vi "Exposure-Save Data.vi"(0 "Params":T3={"Probe Mic Gain"=40.0, "Waveform"=enum."Tone", "CF (kHz)"=1.0, "BW (kHz)"=4.0, "Ear"=enum."Left", "Duration (min)"=0.0, "dB SPL"=120.0, "dB SPL (left)"=0.0}, 5 "SPL Log In":cluster{"t0":dbl, "dt (min)":dbl, "SPL":dbl[][]}, 7 "Spectrum":waveform(dbl)[](graph), 11 "error in (no error)":errorcluster, 13 "State":T2) -> (15 "error out":errorcluster)   [LabVIEW 2020]
uses:
  Typedefs/Exposure Parameters.ctl
  CFTS Main Panel SubVIs/CFTS-Experiment State.ctl
  epl-vi-lib/Utility VIs/Math VIs/LinSpace (x0-dx-npts).vi
  epl-vi-lib/Utility VIs/Array Manipulation VIs/Array-Dimensions (2D).vi
panel:
  in  "Noise Exposure Log File":T1
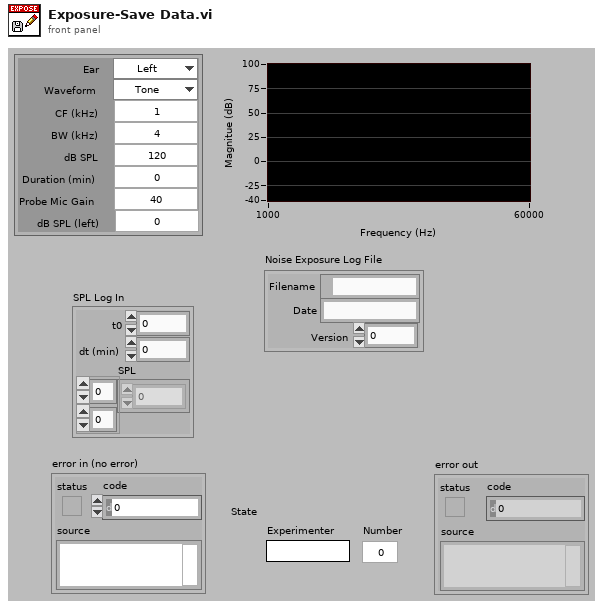
[diagram p1: front panel]
types:
  T1 = cluster{"Filename":path, "Date":string, "Version":i32}
  T2 = typedef "CFTS-Experiment State.ctl" = cluster{"Experimenter":string, "Number":u32, "Right":string, "Left":string, "Data Folder":path, "State File":path, "Version Info":string, "End Exposure Time":dbl, "Exposure Duration":string, "Run #":cluster{"CAP":i16, "ABR":i16, "DP":i16, "VsEP":i16, "MeasSeq":i16, "SubSeq":i16, "SFOAE":i16}}
  T3 = typedef "Exposure Parameters.ctl" = cluster{"Probe Mic Gain":dbl, "Waveform":enum16{"Tone", "Noise"}, "CF (kHz)":dbl, "BW (kHz)":dbl, "Ear":enum16{"Right", "Left", "Binaural"}, "Duration (min)":dbl, "dB SPL":dbl, "dB SPL (left)":dbl}
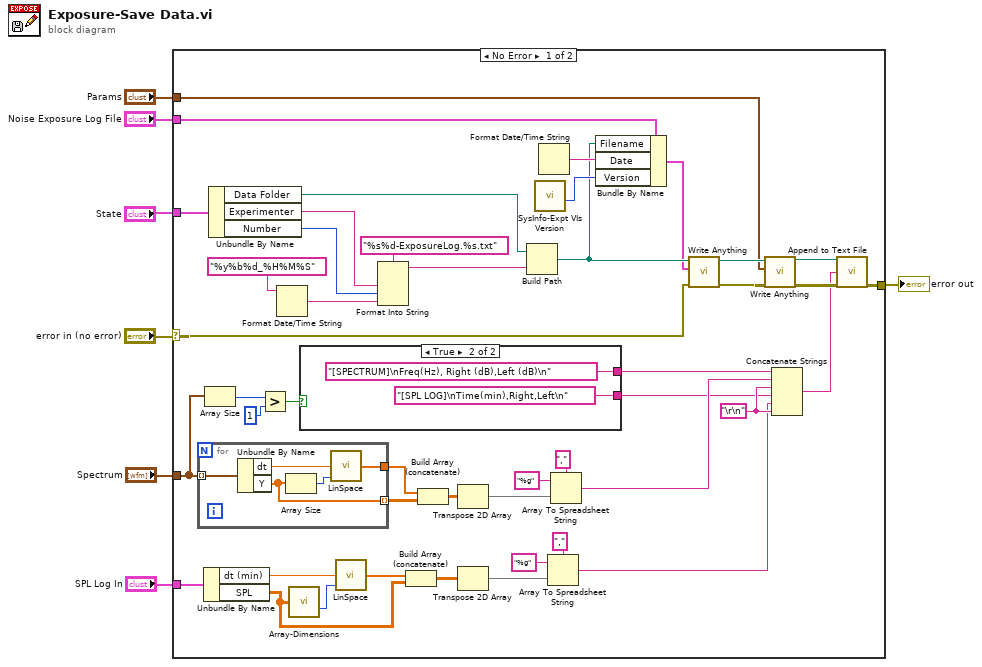
[diagram p0: block diagram]
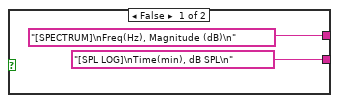
[diagram p2: hidden frame]
diagram:
  n1 = case shown="No Error" "error in (no error)" {
    selector: "error in (no error)" -> [w39 w62]
    tunnel: [w34 w62] -> w6
    tunnel: "State" -> [w52 _]
    tunnel: "Noise Exposure Log File" -> [w44 _]
    tunnel: "Params" -> [w36 _]
    tunnel: "Spectrum" -> [w32 _]
    tunnel: "SPL Log In" -> [w18 _]
    frame No Error {
      w20 = "\r\n"
      n2 = for {
        tunnel: w32 -> [w59] mode=indexing
        tunnel: [w58] -> w29
        tunnel: [w57] -> w28 mode=indexing
        n3 = Unbundle By Name(w59) -> ("dt"=w61:dbl, "Y"=w57:dbl[])
        n4 = Array Size(array=w57) -> (size(s)=w60:i32)
        n5 = call-poly "LinSpace.vi"("npts"=w60, "dx"=w61) -> ("Array"=w58:dbl[])  [unwired: 2 in, 1 out]
      }
      n6 = Unbundle By Name(w18) -> ("dt (min)"=w17:dbl, "SPL"=w15:dbl[][])
      n7 = Array Size(array=w32) -> (size(s)=w31:i32)
      n8 = Unbundle By Name(w52) -> ("Data Folder"=w46:path, "Experimenter"=w50:string, "Number"=w49:u32)
      n9 = Greater?(x=w31, y=1) -> (0:w22:bool)
      n10 = Format Date/Time String(time format string (%c)="%y%b%d_%H%M%S") -> (date/time string=w47:string)  [unwired: 2 in]
      n11 = call-poly "Array-Dimensions.vi"("2D Array"=w15) -> ("# columns"=w8:i32)  [unwired: 13 in, 1 out]
      n12 = case shown="True" w22 {
        tunnel: ["[SPECTRUM]\nFreq(Hz), Magnitude (dB)\n" "[SPECTRUM]\nFreq(Hz), Right (dB),Left (dB)\n"] -> w23
        tunnel: ["[SPL LOG]\nTime(min), dB SPL\n" "[SPL LOG]\nTime(min),Right,Left\n"] -> w19
        frame False {
        }
        frame True {
        }
      }
      n13 = call-poly "LinSpace.vi"("npts"=w8, "dx"=w17) -> ("Array"=w16:dbl[])  [unwired: 2 in, 1 out]
      n14 = Format Into String(format string="%s%d-ExposureLog.%s.txt", w50, w49, w47) -> (resulting string=w45:string)  [unwired: 2 in, 1 out]
      n15 = Build Array (concatenate)(w16, w15) -> (w12:dbl[][])
      n16 = Build Array (concatenate)(w29, w28) -> (w25:dbl[][])
      n17 = Transpose 2D Array(2D array=w25) -> (transposed array=w10:dbl[][])
      n18 = Transpose 2D Array(2D array=w12) -> (transposed array=w9:dbl[][])
      n19 = Build Path(base path=w46, name or relative path=w45) -> (appended path=w41:path)
      n20 = call "SysInfo-Expt VIs Version.vi"() -> ("Expt VIs Version out"=w42:i32)  [unwired: 11 in]
      n21 = Format Date/Time String() -> (date/time string=w43:string)  [unwired: 3 in]
      n22 = Array To Spreadsheet String(delimiter (Tab)=",", array=w9, 3:"%g" ("format string")) -> (spreadsheet string=w11:string)
      n23 = Array To Spreadsheet String(delimiter (Tab)=",", array=w10, 3:"%g" ("format string")) -> (spreadsheet string=w21:string)
      n24 = Bundle By Name(cluster=w44, "Filename"=w41, "Date"=w43, "Version"=w42) -> (w40:T1)
      n25 = call "Write Anything.vi"("Error In"=w39, "Anything"=w40, "Path (dialog)"=w41) -> ("Error Out"=w38:errorcluster, "Path out"=w37:path)  [unwired: 7 in]
      n26 = call "Write Anything.vi"("Error In"=w38, "Anything"=w36, "Path (dialog)"=w37) -> ("Error Out"=w35:errorcluster, "Path out"=w33:path)  [unwired: 7 in]
      n27 = Concatenate Strings(w23, w21, w20, w19, w11, w20) -> (w24:string)
      n28 = call "Append to Text File.vi"("file path"=w33, "text"=w24, "error in (no error)"=w35) -> ("error out"=w34:errorcluster)  [unwired: 11 in, 1 out]
    }
    frame Error {
    }
  }
  "error out" <- w6
